vi "Waveform Analysis (Events).vi"() -> ()   [LabVIEW 2012]
uses:
  <vilib>/Analysis/2dsp.llb/Real FFT.vi
  <vilib>/Analysis/NI_AALPro.lvlib
panel:
  out "频谱":dbl[](graph)
  out "最小值":dbl
  out "最大值":dbl
  out "时间序列":dbl[](graph)
  in  "获取最大值与最小值":bool
  in  "计算FFT":bool
  in  "获取时间序列":bool
  in  "停止":bool
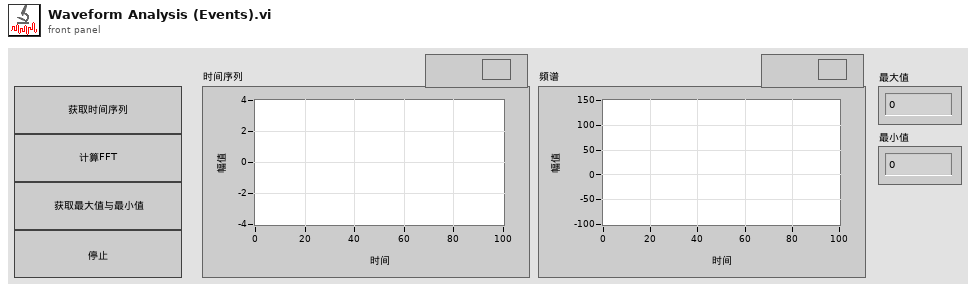
[diagram p1: front panel]
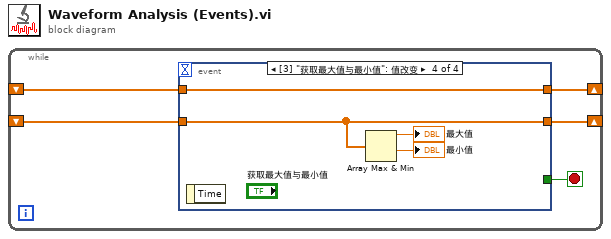
[diagram p0: block diagram]
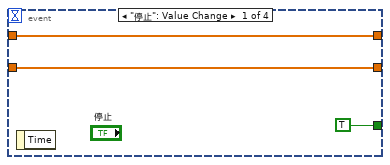
[diagram p2: hidden frame]
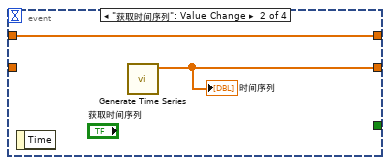
[diagram p3: hidden frame]
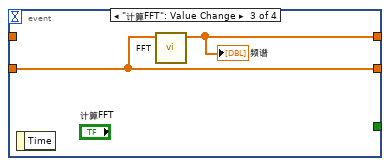
[diagram p4: hidden frame]
diagram:
  n1 = while {
    shift-right: [w4] -> _
    shift-left: _ -> [w3]
    shift-right: [w2] -> _
    shift-left: _ -> [w1]
    stop <- w5 stop-if-true
    n2 = event shown="[3] \"获取最大值与最小值\": 值改变" {
      selector: _ -> [_ _ _ _]
      dyn-events: _ -> [_ _ _ _]
      timeout: _ -> [_ _ _ _]
      tunnel: [TRUE _ _ _] -> w5
      tunnel: [w7 w9 w12 w15] -> w4
      tunnel: w3 -> [w7 _ w12 w15]
      tunnel: [w6 w10 w11 w16] -> w2
      tunnel: w1 -> [w6 w10 _ w16]
      event "停止": Value Change {
        n3 = event-data ("事件数据节点")() -> ()  [unwired: 1 in, 1 out]
      }
      event "获取时间序列": Value Change {
        n4 = event-data ("事件数据节点")() -> ()  [unwired: 1 in, 1 out]
        n5 = call "Generate Time Series.vi"() -> ("时间序列"=w9:dbl[])  [unwired: 11 in]
        "时间序列" <- w9
      }
      event "计算FFT": Value Change {
        n6 = event-data ("事件数据节点")() -> ()  [unwired: 1 in, 1 out]
        n7 = call-poly <vilib>:"FFT.vi"("X"=w12) -> ("FFT {X}"=w11:cdb[])  [unwired: 9 in, 1 out]
        "频谱" <- w11
      }
      event "获取最大值与最小值": Value Change {
        n8 = event-data ("事件数据节点")() -> ()  [unwired: 1 in, 1 out]
        n9 = Array Max & Min ("数组最大值与最小值")(array=w15) -> (max value=→"最大值":dbl, min value=→"最小值":dbl)  [unwired: 2 out]
      }
    }
  }
